vi "Set Pressure Control Mode.vi"(8 "error in":errorcluster, 11 "Red-y Read Write CFG in":refnum<class "Red-y Pressure Control CFG.lvclass">) -> (0 "error out":errorcluster, 3 "Red-y Read Write CFG out":refnum<class "Red-y Pressure Control CFG.lvclass">)   [LabVIEW 2023]
uses:
  Red-y Pressure Control CFG.lvclass
  Read Write PE Input.ctl
  <userlib>/_OpenG.lib/lvdata/lvdata.llb/Type Descriptor Enumeration__ogtk.ctl
  Configuration/Configuration JSON/Configuration JSON Base/CFG JSON.lvclass/CFG JSON.ctl
  1a6763ef-90d6-41fc-ade0-2426224078ff.vi
  <vilib>/JDP Science/JSONtext/Find Item.vi
  <vilib>/JDP Science/JSONtext/Next JSON Value.vi
  <vilib>/JDP Science/JSONtext/String Subset.vi
  <vilib>/JDP Science/JSONtext/Parsing/Advance past next JSON Value (inlined COPY).vi
  <vilib>/JDP Science/JSONtext/Parsing/Advance past whitespace.vi
  <vilib>/JDP Science/JSONtext/Parsing/Advance past String.vi
  <vilib>/JDP Science/JSONtext/Parsing/Advance past Number.vi
  <vilib>/JDP Science/JSONtext/Parsing/Advance past Line Ending.vi
  <vilib>/JDP Science/JSONtext/Parsing/Parse Full Path or Item Name.vi
  <vilib>/JDP Science/JSONtext/Parsing/Advance past Array.vi
  <vilib>/JDP Science/JSONtext/Parsing/Advance past Object.vi
  <vilib>/JDP Science/JSONtext/support/Error Cluster From Code.vi
  <vilib>/JDP Science/JSONtext/Offset/Find Item Locations by Path.vi
  <vilib>/JDP Science/JSONtext/JSON text to Variant.vi
  <vilib>/JDP Science/JSONtext/LVClass Serializer/JSONtext LVClass Serializer.lvclass
  <userlib>/_OpenG.lib/lvdata/lvdata.llb/openg_variant.lvlib
  Configuration/Configuration JSON/Configuration JSON Base/CFG JSON.lvclass
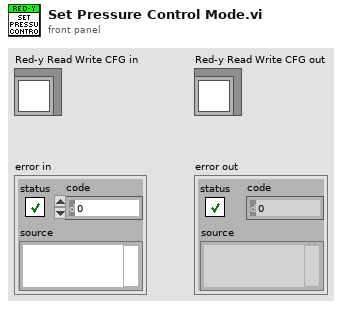
[diagram p1: front panel]
types:
  T1 = typedef "openg_variant.lvlib/Type Descriptor Enumeration__ogtk.ctl" = enum8{"<Null>", "I8", "I16", "I32", "I64", "U8", "U16", "U32", "U64", "SGL", "DBL", "EXT", "CSG", "CDB", "CXT", "0x0F", "0x10", "0x11", "0x12", "0x13", "0x14", "Enum U8", "Enum U16", "Enum U32", "Enum U64", "SGL PQ", "DBL PQ", "EXT PQ", "CSG PQ", "CDB PQ", "CXT PQ", "0x1F", "0x20", "Boolean", "0x22", "0x23", "0x24", "0x25", "0x26", "0x27", "0x28", "0x29", "0x2A", "0x2B", "0x2C", "0x2D", "0x2E", "0x2F", "String", "0x31", "Path", "Pict", "0x34", "0x35", "0x36", "DAQ", "0x38", "0x39", "0x3A", "0x3B", "0x3C", "0x3D", "0x3E", "0x3F", "Array", "0x41", "0x42", "0x43", "0x44", "0x45", "0x46", "0x47", "0x48", "0x49", "0x4A", "0x4B", "0x4C", "0x4D", "0x4E", "0x4F", "Cluster", "0x51", "0x52", "Variant", "Waveform", "0x55", "0x56", "0x57", "0x58", "0x59", "0x5A", "0x5B", "0x5C", "0x5D", "0x5E", "Fixed Point", "0x60", "0x61", "0x62", "0x63", "0x64", "0x65", "0x66", "0x67", "0x68", "0x69", "0x6A", "0x6B", "0x6C", "0x6D", "0x6E", "0x6F", "Refnum", "0x71", "0x72", "Set Collection", "Map Collection"}
  T2 = typedef "Read Write PE Input.ctl" = cluster{"Action":enum16{"Write", "Read"}, "Register":u16, "Type":T1, "Data":variant}
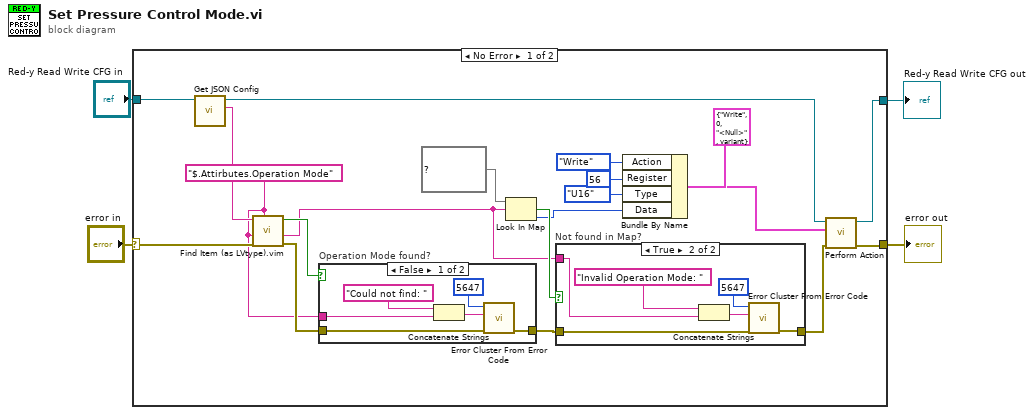
[diagram p0: block diagram]
diagram:
  n1 = case shown="No Error" "error in" {
    selector: "error in" -> [w15 w40]
    tunnel: [w19 w40] -> w3
    tunnel: [w17 w39] -> w1
    tunnel: "Red-y Read Write CFG in" -> [w18 w39]
    frame No Error {
      w11 = "$.Attirbutes.Operation Mode" ("$Path or Item Name")
      n2 = call "Get JSON Config.vi"("CFG Base in"=w18) -> ("<JSON>Config>"=w14:string, "CFG Base out"=w16:refnum<class "Red-y Pressure Control CFG.lvclass">)  [unwired: 9 in]
      n3 = call "Find Item (as LVtype).vim"("$Path or Item Name"=w11, "error in (no error)"=w15, "Data Type and Default Value"=w11, "JSON"=w14) -> ("error out"=w13:errorcluster, "Data"=w6:string, "Found"=w12:bool)  [unwired: 4 in, 1 out]
      n4 = case "Operation Mode found?" shown="False" w12 {
        tunnel: w13 -> [w30 w31]
        tunnel: [w25 w31] -> w9
        tunnel: w11 -> [w26 _]
        frame False {
          n5 = Concatenate Strings("Could not find: " ("string"), w26) -> (w28:string)
          n6 = call <vilib>:"Error Cluster From Error Code.vi"("error in (no error)"=w30, "error message (\"\")"=w28, "error code (0)"=5647) -> ("error out"=w25:errorcluster)  [unwired: 6 in]
        }
        frame True {
        }
      }
      n7 = Look In Map(map=map{string, u8} {"Analog Setpoint"=2, "Back Pressure Control"=6, "Digital Setpoint"=1, "Flow Automatic"=0, "Pressure Control"=5} ("map out"), key=w6) -> (key not found?=w7:bool, value=w5:u8)  [unwired: 1 in]
      n8 = case "Not found in Map?" shown="True" w7 {
        tunnel: w9 -> [w32 w35]
        tunnel: [w32 w34] -> w8
        tunnel: w6 -> [_ w33]
        frame False {
        }
        frame True {
          n9 = Concatenate Strings("Invalid Operation Mode: " ("string"), w33) -> (w37:string)
          n10 = call <vilib>:"Error Cluster From Error Code.vi"("error in (no error)"=w35, "error message (\"\")"=w37, "error code (0)"=5647) -> ("error out"=w34:errorcluster)  [unwired: 6 in]
        }
      }
      n11 = Bundle By Name(cluster=T2 {"Action"=enum."Write", "Register"=0, "Type"=enum."<Null>", "Data"=variant}, "Action"=enum16{"Write", "Read"}."Write", "Register"=u16 56 ("Register Start Address"), "Type"=Type_Descriptor_Enumeration__ogtk."U16", "Data"=w5) -> (w23:T2)
      n12 = call-dynamic "Perform Action.vi"("error in"=w8, "Input"=w23, "Red-y Read Write CFG in"=w16) -> ("error out"=w19:errorcluster, "Red-y Read Write CFG out"=w17:refnum<class "Red-y Pressure Control CFG.lvclass">)  [unwired: 6 in, 1 out]
    }
    frame Error {
    }
  }
  "error out" <- w3
  "Red-y Read Write CFG out" <- w1
